vi "Target Logger File Writer v2.vi"(5 "State":T5=enum."Accumulate", 7 "Data":T1, 8 "Input Array":dbl[][](array[numeric]), 11 "Array Index":i32) -> (0 "Output Array":dbl[][](array[numeric]), 3 "Array Index Out":i32)   [LabVIEW 2018]
uses:
  Target Logger States.ctl
  Logging Data Cluster.ctl
  Target Logging Control Signals.ctl
  Target Logging Sensors.ctl
  Sensor Data.ctl
panel:
  out "Write Metadata Error":errorcluster
  out "appended path":path
  out "Write Main Error":errorcluster
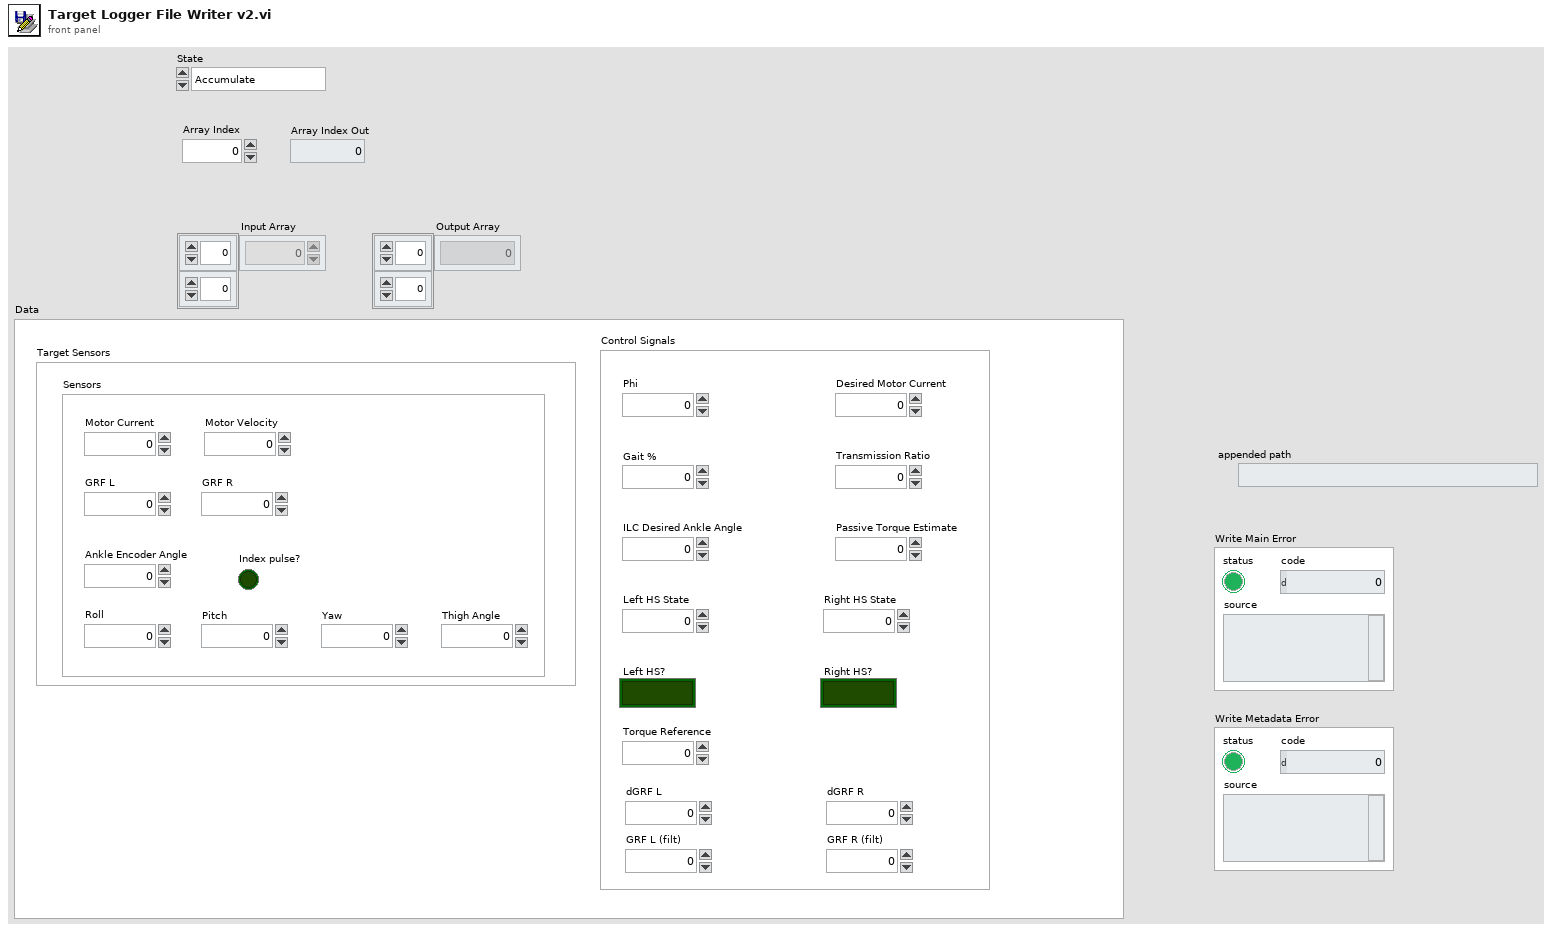
[diagram p1: front panel]
types:
  T1 = typedef "Logging Data Cluster.ctl" = cluster{"Control Signals":T2, "Target Sensors":T3}
  T2 = typedef "Target Logging Control Signals.ctl" = cluster{"Phi":dbl, "Gait %":dbl, "ILC Desired Ankle Angle":dbl, "Desired Motor Current":dbl, "Transmission Ratio":dbl, "Passive Torque Estimate":dbl, "Torque Reference":dbl, "Left HS?":bool, "Left HS State":u32, "Right HS?":bool, "Right HS State":u32, "dGRF L":dbl, "dGRF R":dbl, "GRF L (filt) ":dbl, "GRF R (filt)":dbl}
  T3 = typedef "Target Logging Sensors.ctl" = cluster{"Sensors":T4}
  T4 = typedef "Sensor Data.ctl" = cluster{"Motor Current":dbl, "Motor Velocity":dbl, "Ankle Encoder Angle":dbl, "GRF L":dbl, "GRF R":dbl, "Index pulse?":bool, "Roll":dbl, "Pitch":dbl, "Yaw":dbl, "Thigh Angle":dbl}
  T5 = typedef "Target Logger States.ctl" = enum16{"Idle", "Accumulate", "Write Main", "Write Metadata"}
  T6 = enum16{"open", "open or create", "create or replace", "create", "open (read-only)"}
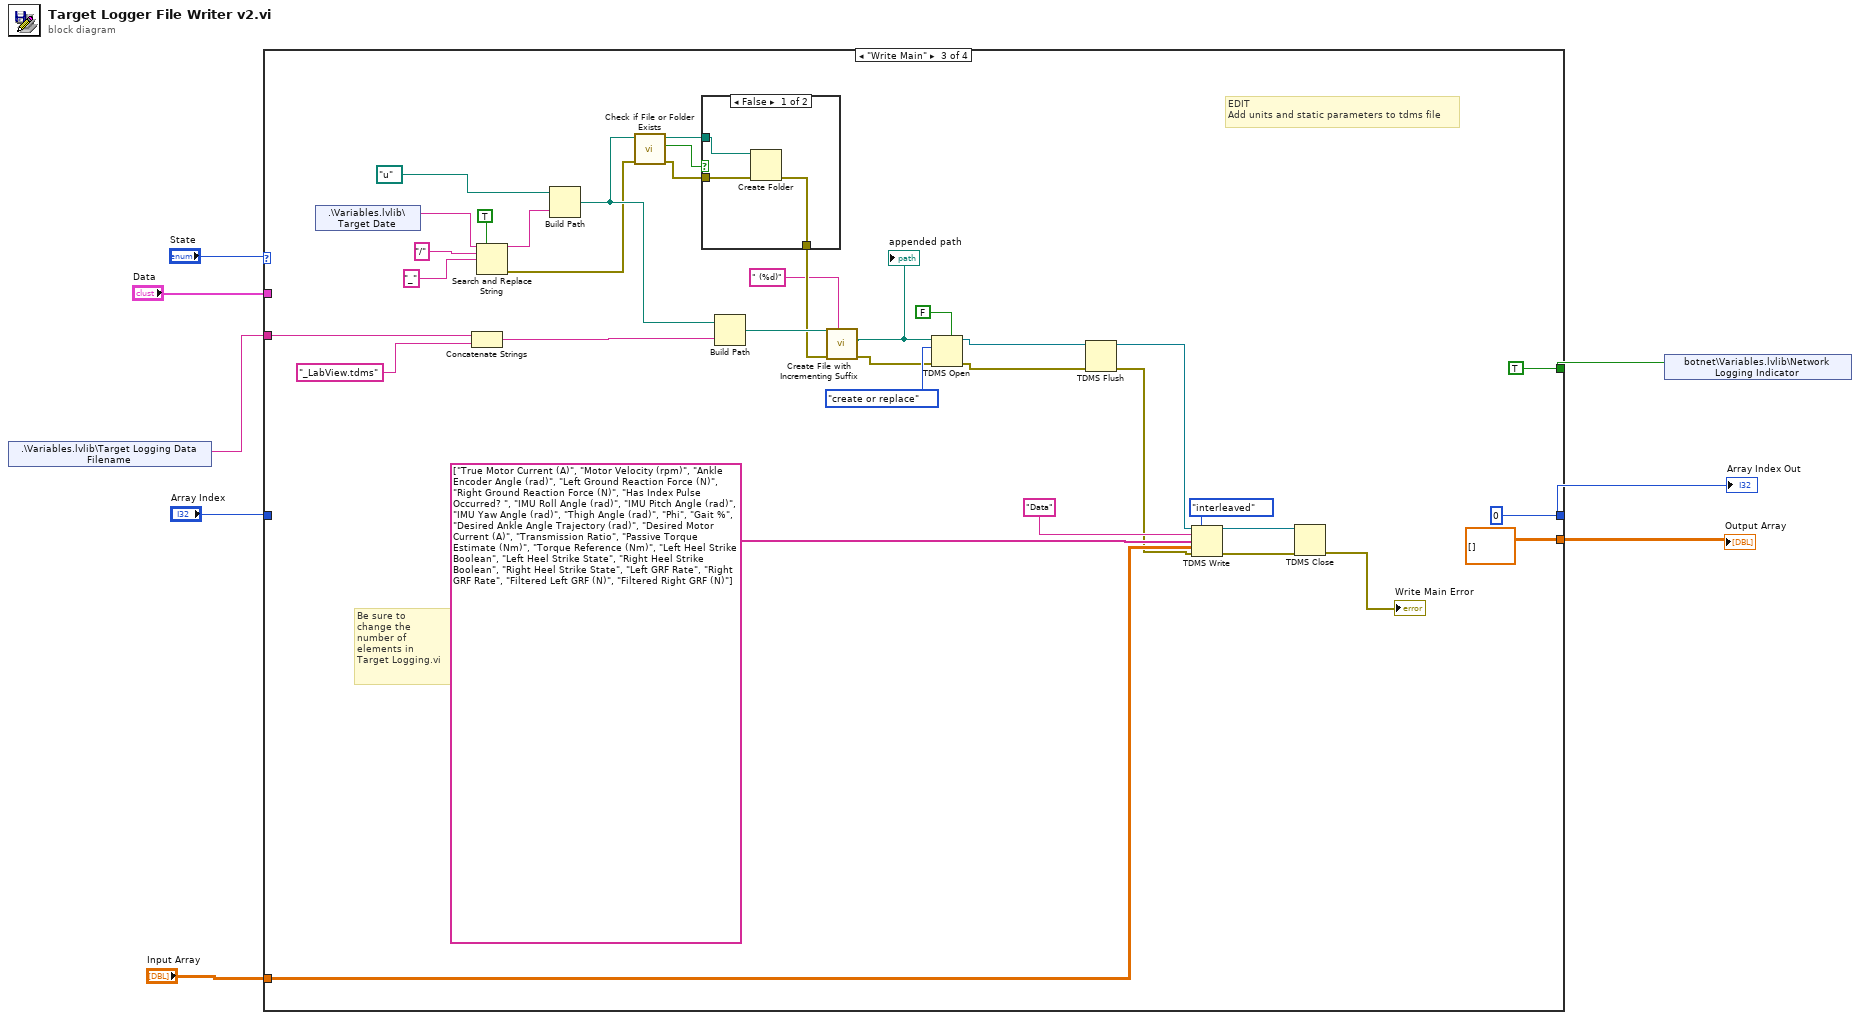
[diagram p0: block diagram]
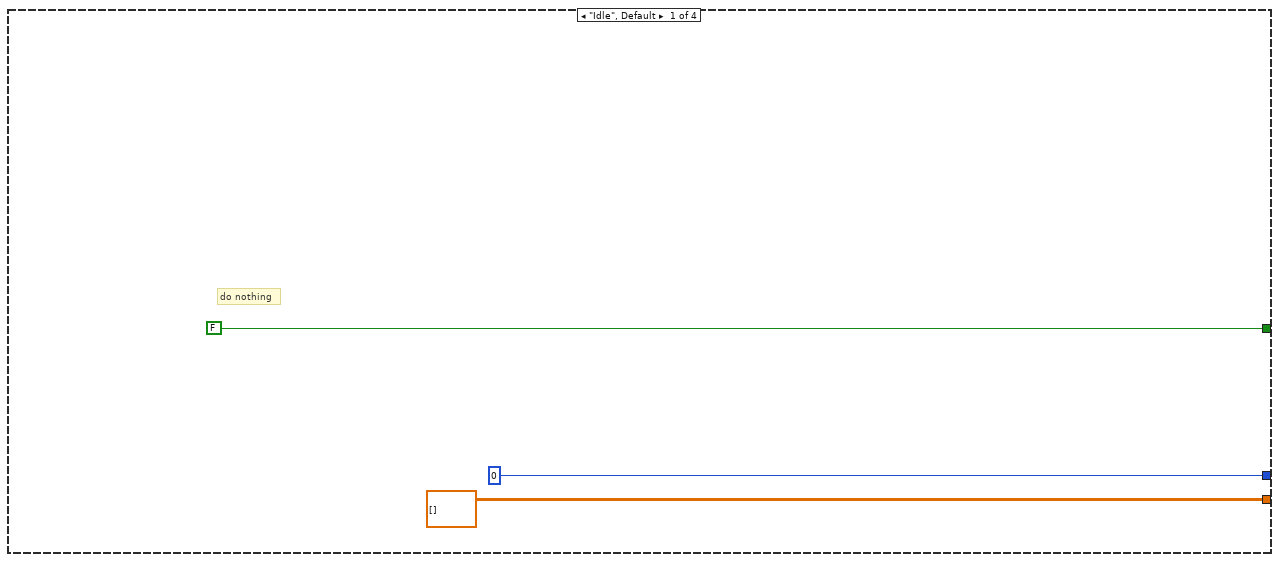
[diagram p2: hidden frame]
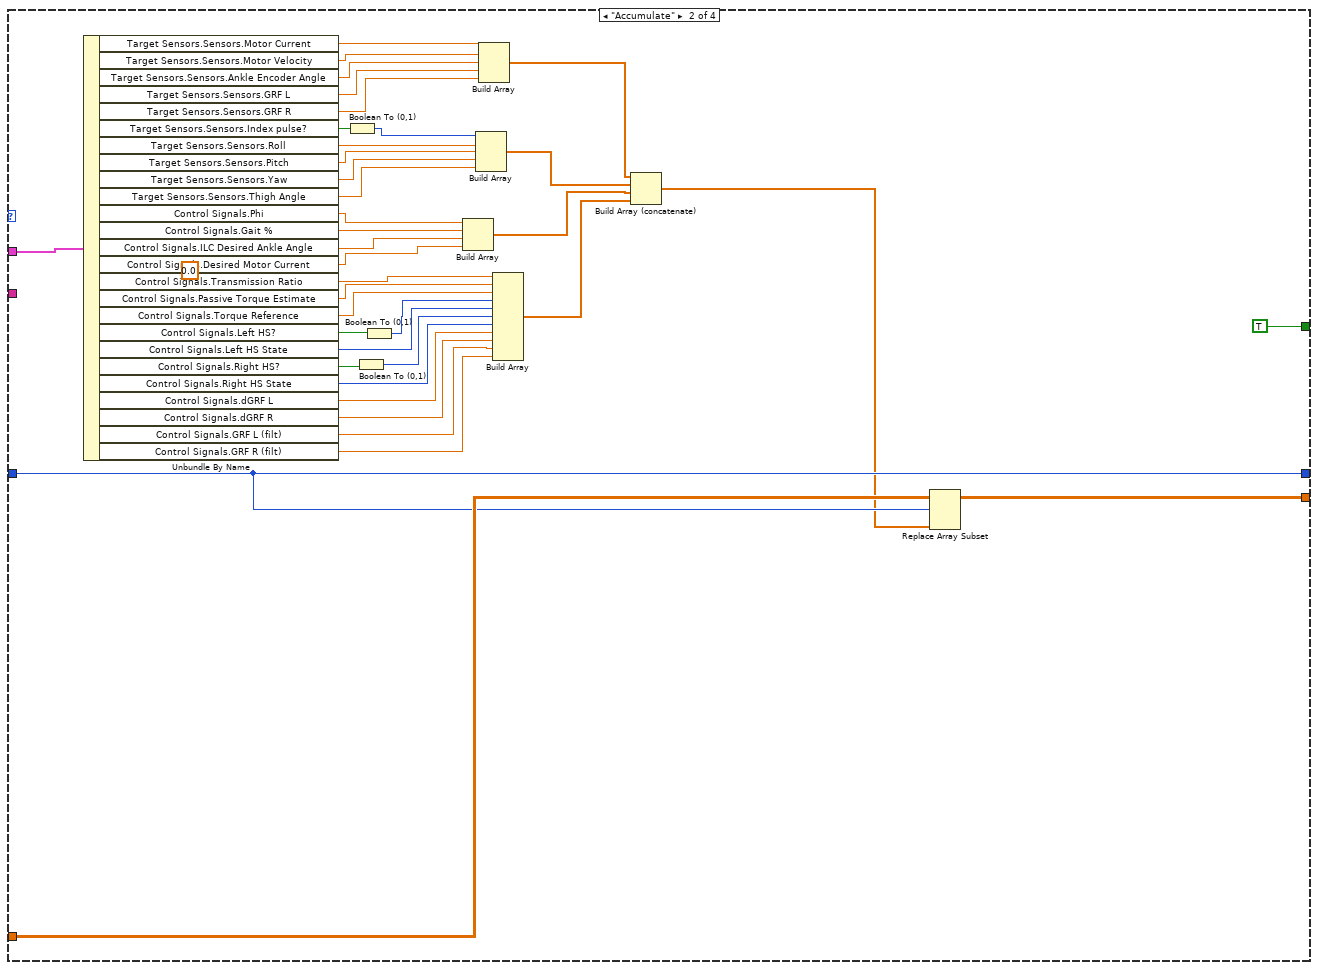
[diagram p3: hidden frame]
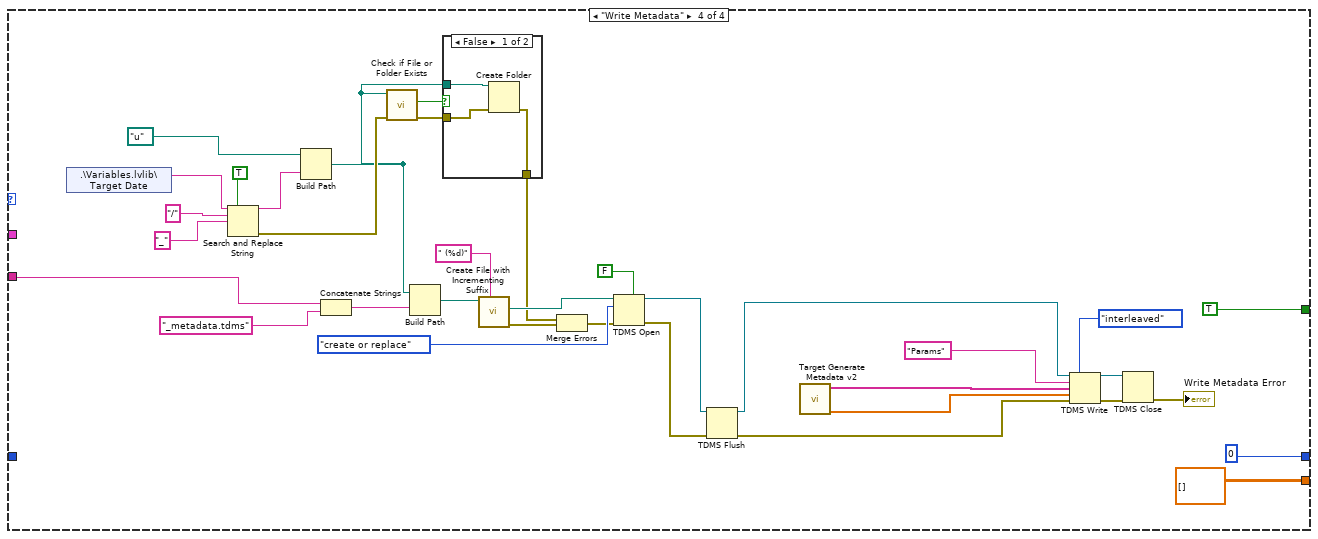
[diagram p5: hidden frame]
diagram:
  n1 = shared-variable ".\\Variables.lvlib\\Target Logging Data Filename"() -> (w1:string)  [unwired: 1 in, 1 out]
  n2 = case shown="\"Write Main\"" "State" {
    tunnel: [dbl[][] [] w48 dbl[][] [] dbl[][] []] -> w4
    tunnel: [FALSE TRUE TRUE TRUE] -> w2
    tunnel: [0 w46 0 0] -> w3
    tunnel: "Input Array" -> [_ w49 w78 _]
    tunnel: "Array Index" -> [_ w46 _ _]
    tunnel: w1 -> [_ _ w75 w120]
    tunnel: "Data" -> [_ w45 _ _]
    frame "Idle", Default {
      # "do nothing"
    }
    frame "Accumulate" {
      (unwired) 0.0 ("element")
      n3 = Unbundle By Name(w45) -> ("Target Sensors.Sensors.Motor Current"=w40:dbl, "Target Sensors.Sensors.Motor Velocity"=w39:dbl, "Target Sensors.Sensors.Ankle Encoder Angle"=w38:dbl, "Target Sensors.Sensors.GRF L"=w37:dbl, "Target Sensors.Sensors.GRF R"=w36:dbl, "Target Sensors.Sensors.Index pulse?"=w35:bool, "Target Sensors.Sensors.Roll"=w33:dbl, "Target Sensors.Sensors.Pitch"=w32:dbl, "Target Sensors.Sensors.Yaw"=w31:dbl, "Target Sensors.Sensors.Thigh Angle"=w30:dbl, "Control Signals.Phi"=w27:dbl, "Control Signals.Gait %"=w44:dbl, "Control Signals.ILC Desired Ankle Angle"=w26:dbl, "Control Signals.Desired Motor Current"=w25:dbl, "Control Signals.Transmission Ratio"=w23:dbl, "Control Signals.Passive Torque Estimate"=w24:dbl, "Control Signals.Torque Reference"=w22:dbl, "Control Signals.Left HS?"=w20:bool, "Control Signals.Left HS State"=w19:u32, "Control Signals.Right HS?"=w18:bool, "Control Signals.Right HS State"=w16:u32, "Control Signals.dGRF L"=w15:dbl, "Control Signals.dGRF R"=w14:dbl, "Control Signals.GRF L (filt)"=w13:dbl, "Control Signals.GRF R (filt)"=w12:dbl)
      n4 = Boolean To (0,1)(Boolean=w35) -> (0, 1=w34:i16)
      n5 = Boolean To (0,1)(Boolean=w18) -> (0, 1=w17:i16)
      n6 = Boolean To (0,1)(Boolean=w20) -> (0, 1=w21:i16)
      n7 = Build Array "Build Array"(w27, w44, w26, w25) -> (w43:dbl[])
      n8 = Build Array "Build Array"(w34, w33, w32, w31, w30) -> (w28:dbl[])
      n9 = Build Array "Build Array"(w40, w39, w38, w37, w36) -> (w29:dbl[])
      n10 = Build Array "Build Array"(w23, w24, w22, w21, w19, w17, w16, w15, w14, w13, w12) -> (w42:dbl[])
      n11 = Build Array (concatenate)(w29, w28, w43, w42) -> (w41:dbl[])
      n12 = Replace Array Subset "Replace Array Subset"(array=w49, new element=w41, index (row)=w46) -> (w48:dbl[][])  [unwired: 1 in]
    }
    frame "Write Main" {
      # "Be sure to\nchange the\nnumber of \nelements in\nTarget Logging.vi"
      # "EDIT\nAdd units and static parameters to tdms file"
      n13 = shared-variable ".\\Variables.lvlib\\Target Date"() -> (w64:string)  [unwired: 1 in, 1 out]
      n14 = Concatenate Strings(w75, "_LabView.tdms" ("string")) -> (w65:string)
      n15 = Search and Replace String(replace all?=TRUE ("replace all? (F)"), input string=w64, search string="/", replace string="_" ("replace string (\"\")")) -> (result string=w63:string, error out=w58:errorcluster)  [unwired: 4 in, 2 out]
      n16 = Build Path(base path=path "u:/", name or relative path=w63) -> (appended path=w59:path)
      n17 = call <vilib>:"Check if File or Folder Exists.vi"("error in (no error)"=w58, "path"=w59) -> ("error out"=w55:errorcluster, "file or folder exists?"=w57:bool, "dup path"=w56:path)  [unwired: 7 in]
      n18 = case shown="False" w57 {
        tunnel: w56 -> [w87 _]
        tunnel: w55 -> [w86 w88]
        tunnel: [w85 w88] -> w51
        frame False {
          n19 = Create Folder(path (use dialog)=w87, error in=w86) -> (error out=w85:errorcluster)  [unwired: 1 in, 2 out]
        }
        frame True {
        }
      }
      n20 = Build Path(base path=w59, name or relative path=w65) -> (appended path=w52:path)
      n21 = call <vilib>:"Create File with Incrementing Suffix.vi"("format string (\" (%d)\")"=" (%d)" ("format string (\" (%d)\")"), "error in (no error)"=w51, "file path"=w52) -> ("error out"=w54:errorcluster, "actual path"=w53:path)  [unwired: 6 in, 1 out]
      "appended path" <- w53
      n22 = TDMS Open(5:FALSE ("create index file? (T)"), 8:w54, 10:T6."create or replace" ("operation (0:open)"), 11:w53) -> (0:w70:errorcluster, 3:w68:refnum<k34>)  [unwired: 3 in]
      n23 = TDMS Flush(4:w70, 7:w68) -> (0:w69:errorcluster, 3:w67:refnum<k34>)
      n24 = TDMS Write(0:w67, 1:enum16{"decimated", "interleaved"}."interleaved" ("data layout (0:decimated)"), 5:"Data" ("group name in (Untitled)"), 7:string[] ["True Motor Current (A)", "Motor Velocity (rpm)", "Ankle Encoder Angle (rad)", "Left Ground Reaction Force (N)", "Right Ground Reaction Force (N)", "Has Index Pulse Occurred? ", "IMU Roll Angle (rad)", "IMU Pitch Angle (rad)", "IMU Yaw Angle (rad)", "Thigh Angle (rad)", "Phi", "Gait %", "Desired Ankle Angle Trajectory (rad)", "Desired Motor Current (A)", "Transmission Ratio", "Passive Torque Estimate (Nm)", "Torque Reference (Nm)", "Left Heel Strike Boolean", "Left Heel Strike State", "Right Heel Strike Boolean", "Right Heel Strike State", "Left GRF Rate", "Right GRF Rate", "Filtered Left GRF (N)", "Filtered Right GRF (N)"] ("channel name(s) in (Untitled)"), 9:w78, 11:w69) -> (4:w83:refnum<k34>, 15:w73:errorcluster)  [unwired: 2 out]
      n25 = TDMS Close(8:w73, 11:w83) -> (0:→"Write Main Error":errorcluster)  [unwired: 1 out]
    }
    frame "Write Metadata" {
      n26 = shared-variable ".\\Variables.lvlib\\Target Date"() -> (w104:string)  [unwired: 1 in, 1 out]
      n27 = Search and Replace String(replace all?=TRUE ("replace all? (F)"), input string=w104, search string="/", replace string="_" ("replace string (\"\")")) -> (result string=w103:string, error out=w99:errorcluster)  [unwired: 4 in, 2 out]
      n28 = Build Path(base path=path "u:/", name or relative path=w103) -> (appended path=w97:path)
      n29 = Concatenate Strings(w120, "_metadata.tdms" ("string")) -> (w106:string)
      n30 = call <vilib>:"Check if File or Folder Exists.vi"("error in (no error)"=w99, "path"=w97) -> ("error out"=w96:errorcluster, "file or folder exists?"=w98:bool)  [unwired: 7 in, 1 out]
      n31 = Build Path(base path=w97, name or relative path=w106) -> (appended path=w94:path)
      n32 = case shown="False" w98 {
        tunnel: w97 -> [w126 _]
        tunnel: w96 -> [w125 w127]
        tunnel: [w124 w127] -> w91
        frame False {
          n33 = Create Folder(path (use dialog)=w126, error in=w125) -> (error out=w124:errorcluster)  [unwired: 1 in, 2 out]
        }
        frame True {
        }
      }
      n34 = call <vilib>:"Create File with Incrementing Suffix.vi"("format string (\" (%d)\")"=" (%d)" ("format string (\" (%d)\")"), "file path"=w94) -> ("error out"=w90:errorcluster, "actual path"=w93:path)  [unwired: 7 in, 1 out]
      n35 = Merge Errors(w91, w90) -> (w92:errorcluster)
      n36 = TDMS Open(5:FALSE ("create index file? (T)"), 8:w92, 10:T6."create or replace" ("operation (0:open)"), 11:w93) -> (0:w110:errorcluster, 3:w108:refnum<k34>)  [unwired: 3 in]
      n37 = TDMS Flush(4:w110, 7:w108) -> (0:w109:errorcluster, 3:w107:refnum<k34>)
      n38 = call "Target Generate Metadata v2.vi"() -> ("Data"=w113:dbl[], "channel name(s)"=w114:string[])  [unwired: 10 in]
      n39 = TDMS Write(0:w107, 1:enum16{"decimated", "interleaved"}."interleaved" ("data layout (0:decimated)"), 5:"Params" ("group name in (Untitled)"), 7:w114, 9:w113, 11:w109) -> (4:w117:refnum<k34>, 15:w111:errorcluster)  [unwired: 2 out]
      n40 = TDMS Close(8:w111, 11:w117) -> (0:→"Write Metadata Error":errorcluster)  [unwired: 1 out]
    }
  }
  "Output Array" <- w4
  "Array Index Out" <- w3
  n41 = shared-variable "botnet\\Variables.lvlib\\Network Logging Indicator"(w2) -> ()  [unwired: 1 in, 1 out]
